vi "FPGA VI_Simulated_WithNoise_Example.vi"() -> ()   [LabVIEW 2019]
uses:
  Types/Injection.Timing.ctl
  Types/Injection.Core.Settings.ctl
  Types/Injection.Global.Settings.ctl
  Types/Injection.Mux.State.ctl
  <vilib>/Platform/TimedLoop/XDataNode/timing_clust.ctl
  <vilib>/Platform/TimedLoop/XDataNode/nitl_modes.ctl
  <vilib>/Platform/TimedLoop/XDataNode/wakeup.ctl
  Types/Injection.Core.Internal.Settings.ctl
  <vilib>/rvi/DataTransferAndStorage/Container/Common/niFpgaContainerGetUniqueNameForEmu.vi
  <vilib>/rvi/DataTransferAndStorage/Container/Common/niFpgaContainerSetEmuInfo.vi
  <vilib>/rvi/eio/common/nirviEmuReportErrorAndStop.vi
  <vilib>/rvi/Emulation/niFpgaGetClockAttributes.vi
  <vilib>/rvi/Emulation/niFpgaSctlEmulationGetInTimedLoop.vi
  <vilib>/rvi/Emulation/niFpgaEmulationReportErrorSimple.vi
  <vilib>/rvi/Memory/Memory_Emulation/nirvimemoryFastEmulation.vi
  <vilib>/rvi/Memory/Memory_Emulation/nirvimemoryEmulation.vi
  <vilib>/rvi/Emulation/niFpgaEmulationIsFPGAContextNoSignature.vi
  <vilib>/rvi/Emulation/niFpgaProcessEmulError.vi
  <vilib>/rvi/errors/nirviReportUnexpectedCaseInternalError (U32).vi
  <vilib>/rvi/Emulation/niFpgaCriticalErrorInLSC.vi
  <vilib>/rvi/DataTransferAndStorage/Container/Common/niFpgaContainerExecOnDevCompGetState.vi
  <vilib>/rvi/errors/niFpgaSetErrorForExecOnDevCompSimple.vi
  <vilib>/rvi/FIFO/Fifo_Resource/nirvififoEmulationSetSize.vi
  <vilib>/rvi/FIFO/Fifo_Resource/nirviFifoEmulationQueueMgr.vi
  <instcachedir>/0/nirviFifoEmulationQueueMgr_E5CAEC123FF24DC58D834DCA3CDAA9B5.lvgen/nirviFifoEmulationQueueMgr_E5CAEC123FF24DC58D834DCA3CDAA9B5_002.vi
  <vilib>/rvi/FIFO/Fifo_Resource/nirvififoEmulationDetermineInputValidOut.vi
  <vilib>/rvi/FIFO/Fifo_Resource/nirvififoEmulationCreateLock.vi
  <vilib>/rvi/FIFO/Fifo_Resource/nirvififoEmulationObtainLock.vi
  <vilib>/rvi/FIFO/Fifo_Resource/nirvififoEmulationReleaseLock.vi
  <vilib>/rvi/occurrence/nirviWaitOnOccurrenceBase.vi
  <vilib>/rvi/errors/nirviReportUnexpectedCaseInternalError.vi
  <vilib>/Utility/error.llb/Clear Errors.vi
  <vilib>/rvi/interface/RandomDataEmulation/niFpgaRandomDataHandleErrors.vi
  <instcachedir>/0/nirviFifoEmulationQueueMgr_E5CAEC123FF24DC58D834DCA3CDAA9B5.lvgen/nirviFifoEmulationQueueMgr_E5CAEC123FF24DC58D834DCA3CDAA9B5_001.vi
  <vilib>/rvi/LocalResourceManager/LocalResourceManager.xnode
  <vilib>/rvi/DataTransferAndStorage/Container/XNode/niFpgaContainer.xnode
  <vilib>/Platform/TimedLoop/XDataNode/XDataNode.xnode
  <vilib>/rvi/FIFO/Fifo_Resource/niFpgaFifoEmulationRefIn.vi
  <vilib>/rvi/interface/RandomDataEmulation/nirviRandomDataFpgaReadWriteTemplate.vi
  <vilib>/Platform/TimedLoop/XDataNode/XDNodeRunTimeDep.lvlib
panel:
  out "Intermediate FIFO Write Timeout":bool
  in  "Settings.Global.Injectors":T1={"Enable?"=FALSE, "Initial Voltage Threshold"=12.0, "Event Dwell Limit"=2000, "Voltage Gain"=1.0, "Current Gain"=1.0, "Filter Samples"=5, "Pretrigger Samples"=5, "Active Edge"=TRUE}
  in  "Settings.Index0.Injectors.Injector0":T2
  in  "Settings.Index1.Injectors.Injector1":T2
  in  "Settings.Index2.Injectors.Injector2":T2
  in  "Settings.Index3.Injectors.Injector3":T2
  in  "Settings.Index4.Injectors.Injector4":T2
  in  "Settings.Index5.Injectors.Injector5":T2
  in  "Settings.Timing":T3={"Injection Sample Period (Ticks)"=80}
  out "Acqusition Loop Ticks":u32
  in  "Settings.DMA":cluster{"# of Injectors":u8}={"# of Injectors"=6}
  out "Host DMA Out?":bool
  out "Intermediate Time Out?":bool
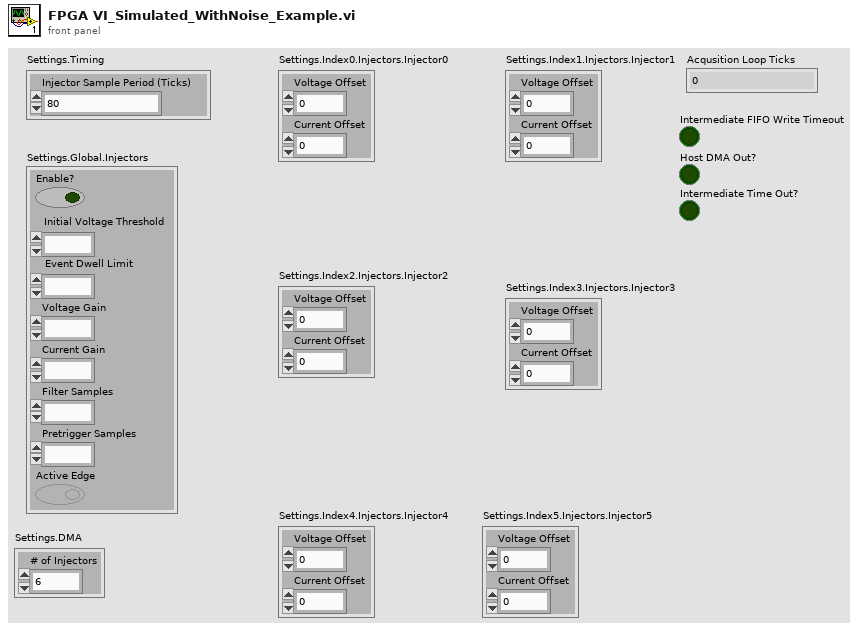
[diagram p1: front panel]
types:
  T1 = typedef "Injection.Global.Settings.ctl" = cluster{"Enable?":bool, "Initial Voltage Threshold":fxp<+/-,32,8>, "Event Dwell Limit":u16, "Voltage Gain":fxp<+/-,32,8>, "Current Gain":fxp<+/-,32,8>, "Filter Samples":u8, "Pretrigger Samples":u8, "Active Edge":bool}
  T2 = typedef "Injection.Core.Settings.ctl" = cluster{"Voltage Offset":fxp<+/-,32,8>, "Current Offset":fxp<+/-,32,8>}
  T3 = typedef "Injection.Timing.ctl" = cluster{"Injection Sample Period (Ticks)":u32}
  T4 = cluster{"Data.Samples":u32, "Injection.Period":u32, "Injector.Index":u8, "Iteration":u32}
  T5 = typedef "Injection.Mux.State.ctl" = enum8{"Wait on Transfer", "Transfer Injector Index", "Transfer # of Samples", "Transfer Injection Period", "Transfer Data Samples"}
  T6 = typedef "XDNodeRunTimeDep.lvlib/timing_clust.ctl" = cluster{"Expected End [f-1]":u64, "Actual End [f-1]":u64, "Finished Late? [f-1]":bool, "Expected End [i-1]":u64, "Actual End [i-1]":u64, "Finished Late? [i-1]":bool, "Expected Start [i]":u64, "Actual Start [i]":u64, "Expected Start [f]":u64, "Actual Start [f]":u64, "Source Name":string, "Structure Name":string, "Period":i64, "Deadline":i64, "Offset":i64, "Start":i64, "Priority":i32, "Timeout":i32, "Mode":T7, "Wakeup Reason":T8, "Error":errorcluster, "Source Type":string, "Secondary Source Type":string, "Global End Time":u64, "Global Start Time":u64, "Frame Duration":u64, "Iteration Duration":u64, "Assigned CPU":i32, "I/O Scan Engine Mode":u32}
  T7 = typedef "XDNodeRunTimeDep.lvlib/nitl_modes.ctl" = enum32{"No Change", "Process missed periods, maintain original phase", "Discard missed periods, maintain original phase", "Process missed periods, ignore original phase", "Discard missed periods, ignore original phase"}
  T8 = typedef "XDNodeRunTimeDep.lvlib/wakeup.ctl" = enum32{"Normal", "Aborted", "Asynchronous wakeup", "Timing source error", "Timed loop error", "Timeout"}
  T9 = typedef "Injection.Core.Internal.Settings.ctl" = cluster{"Data Buffer FIFO":refnum<k21>, "Capture Complete Trigger FIFO":refnum<k21>}
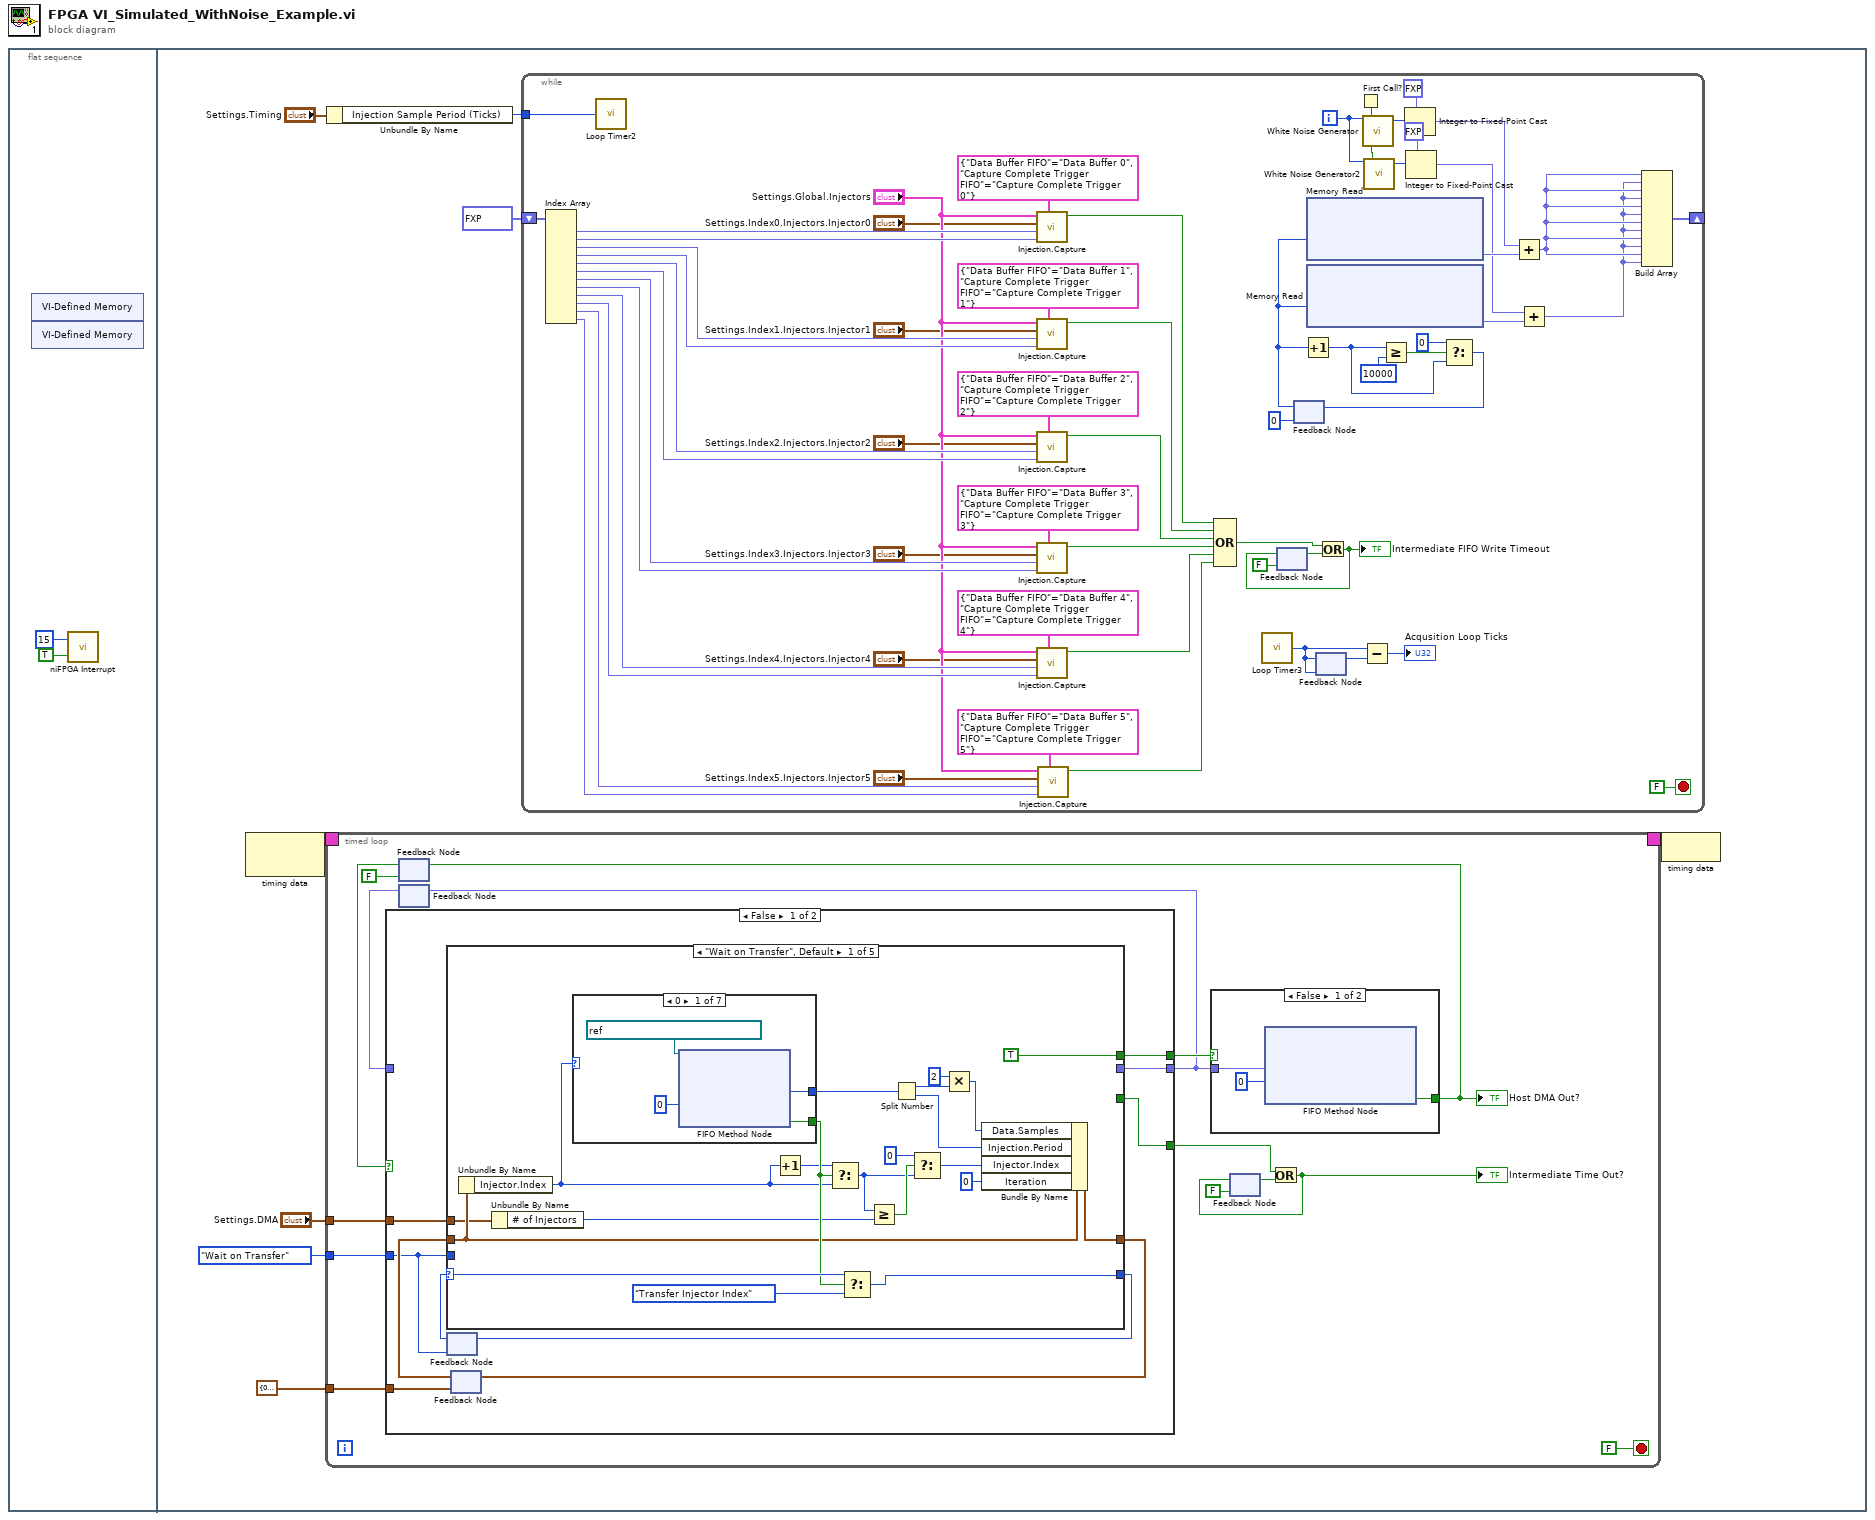
[diagram p0: block diagram]
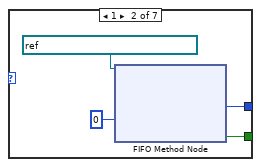
[diagram p2: hidden frame]
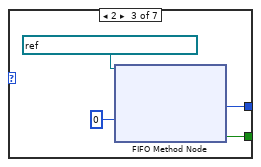
[diagram p3: hidden frame]
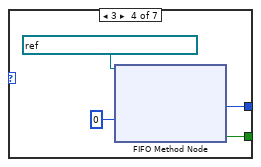
[diagram p4: hidden frame]
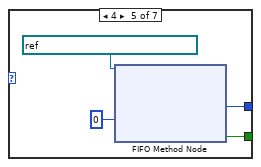
[diagram p5: hidden frame]
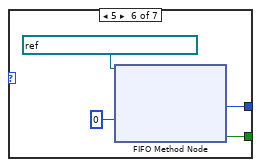
[diagram p6: hidden frame]
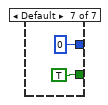
[diagram p7: hidden frame]
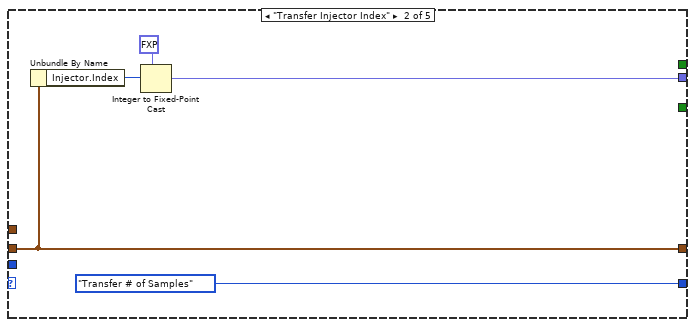
[diagram p8: hidden frame]
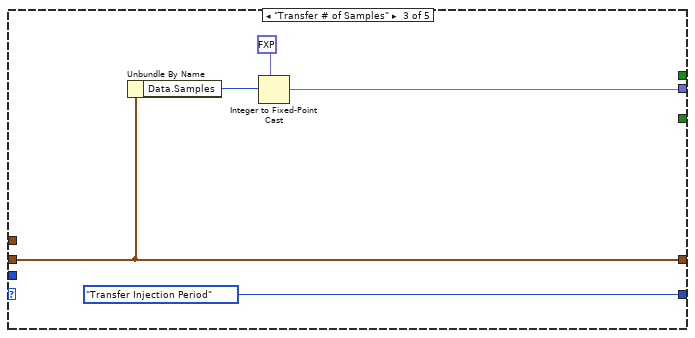
[diagram p9: hidden frame]
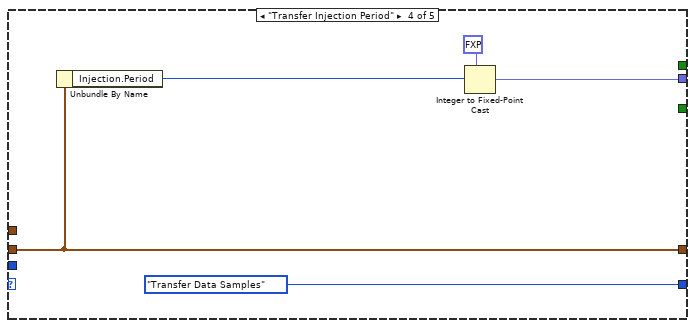
[diagram p10: hidden frame]
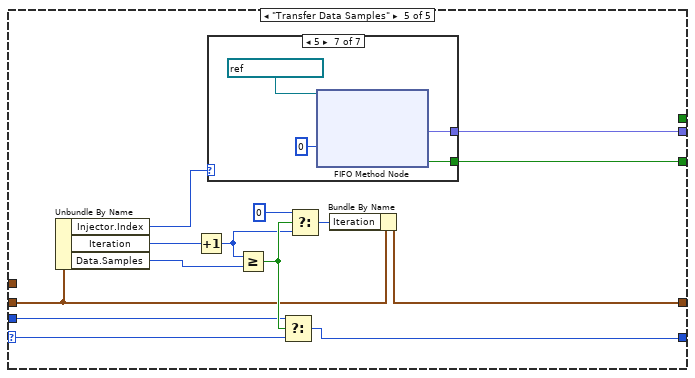
[diagram p11: hidden frame]
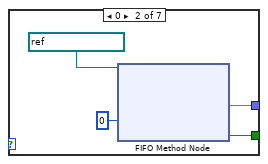
[diagram p13: hidden frame]
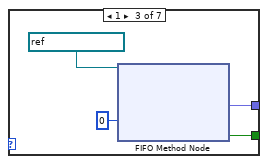
[diagram p14: hidden frame]
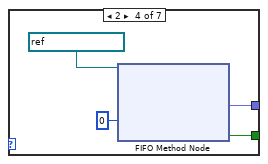
[diagram p15: hidden frame]
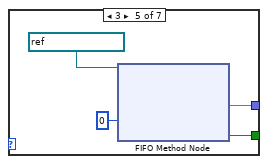
[diagram p16: hidden frame]
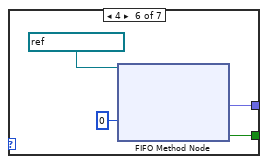
[diagram p17: hidden frame]
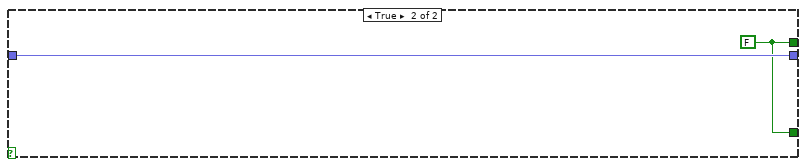
[diagram p18: hidden frame]
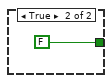
[diagram p19: hidden frame]
diagram:
  n1 = flat-sequence {
    frame #0 {
      n2 = xnode "VI-Defined Memory"() -> ()  [unwired: 1 out]
      n3 = xnode "VI-Defined Memory"() -> ()  [unwired: 1 out]
      n4 = call <vilib>:"niFPGA Interrupt.vi"("Wait Until Cleared (F)"=TRUE, "IRQ Number (0)"=u8 15) -> ()  [unwired: 1 in]
    }
    frame #1 {
      n5 = node-c288() -> (w10:T6)  [unwired: 1 in]
      n6 = timed-loop {
        timing: w10 -> [_]
        timing-out: [_] -> w9
        tunnel: "Settings.DMA" -> [w14]
        tunnel: Injection.Mux.State."Wait on Transfer" -> [w13]
        tunnel: T4 {"Data.Samples"=0, "Injection.Period"=0, "Injector.Index"=0, "Iteration"=0} ("Local.Data") -> [w12]
        stop <- FALSE stop-if-true
        n7 = feedback #1(FALSE ("Timed Out?")) -> (w22:bool)
        n8 = feedback #2() -> (w19:fxp<+/-,32,8>)  [unwired: 1 in]
        n9 = case shown="False" w22 {
          tunnel: [w34 w136] -> w20
          tunnel: [w33 w135] -> w24
          tunnel: w13 -> [w27 _]
          tunnel: [w32 w135] -> w15
          tunnel: w14 -> [w31 _]
          tunnel: w12 -> [w28 _]
          tunnel: w19 -> [_ w136]
          frame False {
            n10 = feedback #3(w27) -> (w26:T5)
            n11 = feedback #4(w28) -> (w29:T4)
            n12 = case shown="\"Wait on Transfer\", Default" w26 {
              selector: w26 -> [w55 _ _ _ w104]
              tunnel: w29 -> [w46 w85 w89 w93 w102]
              tunnel: [w54 w85 w89 w93 w101] -> w30
              tunnel: [w53 Injection.Mux.State."Transfer # of Samples" Injection.Mux.State."Transfer Injection Period" Injection.Mux.State."Transfer Data Samples" w103] -> w25
              tunnel: [_ w84 w88 w95 w100] -> w34
              tunnel: [TRUE _ _ _ _] -> w33
              tunnel: w27 -> [_ _ _ _ w97]
              tunnel: [_ _ _ _ w99] -> w32
              tunnel: w31 -> [w43 _ _ _ _]
              frame "Wait on Transfer", Default {
                n13 = Unbundle By Name(w46) -> ("Injector.Index"=w45:u8)
                n14 = Unbundle By Name(w43) -> ("# of Injectors"=w42:u8)
                n15 = case shown="0" w45 {
                  tunnel: [w58 w62 w66 w70 w74 w78 u64 0 ("Element")] -> w41
                  tunnel: [w57 w61 w65 w69 w73 w77 TRUE ("Timed Out?")] -> w51
                  frame 0 {
                    n16 = xnode ("FIFO Method Node")("Timeout"=0, "FIFO In"=refnum<k21> "Capture Complete Trigger 0") -> ("Element"=w58:u64, "Timed Out?"=w57:bool)  [unwired: 1 out]
                  }
                  frame 1 {
                    n17 = xnode ("FIFO Method Node")("Timeout"=0, "FIFO In"=refnum<k21> "Capture Complete Trigger 1") -> ("Element"=w62:u64, "Timed Out?"=w61:bool)  [unwired: 1 out]
                  }
                  frame 2 {
                    n18 = xnode ("FIFO Method Node")("Timeout"=0, "FIFO In"=refnum<k21> "Capture Complete Trigger 2") -> ("Element"=w66:u64, "Timed Out?"=w65:bool)  [unwired: 1 out]
                  }
                  frame 3 {
                    n19 = xnode ("FIFO Method Node")("Timeout"=0, "FIFO In"=refnum<k21> "Capture Complete Trigger 3") -> ("Element"=w70:u64, "Timed Out?"=w69:bool)  [unwired: 1 out]
                  }
                  frame 4 {
                    n20 = xnode ("FIFO Method Node")("Timeout"=0, "FIFO In"=refnum<k21> "Capture Complete Trigger 4") -> ("Element"=w74:u64, "Timed Out?"=w73:bool)  [unwired: 1 out]
                  }
                  frame 5 {
                    n21 = xnode ("FIFO Method Node")("Timeout"=0, "FIFO In"=refnum<k21> "Capture Complete Trigger 5") -> ("Element"=w78:u64, "Timed Out?"=w77:bool)  [unwired: 1 out]
                  }
                  frame Default {
                  }
                }
                n22 = Increment(x=w45) -> (x+1=w50:u8)
                n23 = Select(t=w50, s=w51, f=w45) -> (s? t:f=w48:u8)
                n24 = Select(t=w55, s=w51, f=Injection.Mux.State."Transfer Injector Index") -> (s? t:f=w53:T5)
                n25 = Greater Or Equal?(x=w48, y=w42) -> (x >= y?=w49:bool)
                n26 = Split Number(x=w41) -> (hi(x)=w40:u32, lo(x)=w39:u32)
                n27 = Select(t=u8 0, s=w49, f=w48) -> (s? t:f=w44:u8)
                n28 = Multiply(x=u32 2, y=w40) -> (x*y=w37:u32)
                n29 = Bundle By Name(cluster=w46, "Data.Samples"=w37, "Injection.Period"=w39, "Injector.Index"=w44, "Iteration"=u32 0) -> (w54:T4)
              }
              frame "Transfer Injector Index" {
                n30 = Unbundle By Name(w85) -> ("Injector.Index"=w86:u8)
                n31 = Integer to Fixed-Point Cast(fixed-point type=fxp<+/-,32,8> 0.0, integer=w86) -> (fixed-point=w84:fxp<+/-,32,8>)
              }
              frame "Transfer # of Samples" {
                n32 = Unbundle By Name(w89) -> ("Data.Samples"=w90:u32)
                n33 = Integer to Fixed-Point Cast(fixed-point type=fxp<+/-,32,8> 0.0, integer=w90) -> (fixed-point=w88:fxp<+/-,32,8>)
              }
              frame "Transfer Injection Period" {
                n34 = Unbundle By Name(w93) -> ("Injection.Period"=w94:u32)
                n35 = Integer to Fixed-Point Cast(fixed-point type=fxp<+/-,32,8> 0.0, integer=w94) -> (fixed-point=w95:fxp<+/-,32,8>)
              }
              frame "Transfer Data Samples" {
                n36 = Unbundle By Name(w102) -> ("Injector.Index"=w110:u8, "Iteration"=w105:u32, "Data.Samples"=w98:u32)
                n37 = Increment(x=w105) -> (x+1=w107:u32)
                n38 = case shown="5" w110 {
                  tunnel: [_ w113 w117 w121 w125 w129 w133] -> w100
                  tunnel: [_ w112 w116 w120 w124 w128 w132] -> w99
                  frame Default {
                  }
                  frame 0 {
                    n39 = xnode ("FIFO Method Node")("Timeout"=0, "FIFO In"=refnum<k21> "Data Buffer 0" ("Voltage FIFO")) -> ("Element"=w113:fxp<+/-,32,8>, "Timed Out?"=w112:bool)  [unwired: 1 out]
                  }
                  frame 1 {
                    n40 = xnode ("FIFO Method Node")("Timeout"=0, "FIFO In"=refnum<k21> "Data Buffer 1" ("Voltage FIFO")) -> ("Element"=w117:fxp<+/-,32,8>, "Timed Out?"=w116:bool)  [unwired: 1 out]
                  }
                  frame 2 {
                    n41 = xnode ("FIFO Method Node")("Timeout"=0, "FIFO In"=refnum<k21> "Data Buffer 2" ("Voltage FIFO")) -> ("Element"=w121:fxp<+/-,32,8>, "Timed Out?"=w120:bool)  [unwired: 1 out]
                  }
                  frame 3 {
                    n42 = xnode ("FIFO Method Node")("Timeout"=0, "FIFO In"=refnum<k21> "Data Buffer 3" ("Voltage FIFO")) -> ("Element"=w125:fxp<+/-,32,8>, "Timed Out?"=w124:bool)  [unwired: 1 out]
                  }
                  frame 4 {
                    n43 = xnode ("FIFO Method Node")("Timeout"=0, "FIFO In"=refnum<k21> "Data Buffer 4" ("Voltage FIFO")) -> ("Element"=w129:fxp<+/-,32,8>, "Timed Out?"=w128:bool)  [unwired: 1 out]
                  }
                  frame 5 {
                    n44 = xnode ("FIFO Method Node")("Timeout"=0, "FIFO In"=refnum<k21> "Data Buffer 5" ("Voltage FIFO")) -> ("Element"=w133:fxp<+/-,32,8>, "Timed Out?"=w132:bool)  [unwired: 1 out]
                  }
                }
                n45 = Greater Or Equal?(x=w107, y=w98) -> (x >= y?=w109:bool)
                n46 = Select(t=w97, s=w109, f=w104) -> (s? t:f=w103:T5)
                n47 = Select(t=u32 0, s=w109, f=w107) -> (s? t:f=w106:u32)
                n48 = Bundle By Name(cluster=w102, "Iteration"=w106) -> (w101:T4)
              }
            }
            n49 = feedback-in #3(w25) -> ()
            n50 = feedback-in #4(w30) -> ()
          }
          frame True {
            w135 = FALSE
          }
        }
        n51 = feedback-in #2(w20) -> ()
        n52 = case shown="False" w24 {
          tunnel: w20 -> [w138 _]
          tunnel: [w137 FALSE ("Timed Out?")] -> w23
          frame False {
            n53 = xnode ("FIFO Method Node")("Element"=w138, "Timeout"=0) -> ("Timed Out?"=w137:bool)  [unwired: 1 in, 1 out]
          }
          frame True {
          }
        }
        "Host DMA Out?" <- w23
        n54 = feedback-in #1(w23) -> ()
        n55 = feedback #5(FALSE ("Timed Out?")) -> (w17:bool)
        n56 = Or(x=w15, y=w17) -> (x .or. y?=w16:bool)
        "Intermediate Time Out?" <- w16
        n57 = feedback-in #5(w16) -> ()
      }
      n58 = Unbundle By Name("Settings.Timing") -> ("Injection Sample Period (Ticks)"=w3:u32)
      n59 = while {
        shift-right: [w156] -> _
        shift-left: fxp<+/-,24,5>[] [0.0, 0.0, 0.0, 0.0, 0.0, 0.0, 0.0, 0.0, 0.0, 0.0, 0.0, 0.0] -> [w186]
        tunnel: w3 -> [w170]
        i -> [w151]
        stop <- FALSE stop-if-true
        n60 = Index Array(array=w186) -> (element #1=w197:fxp<+/-,24,5>, element #2=w198:fxp<+/-,24,5>, element #3=w195:fxp<+/-,24,5>, element #4=w196:fxp<+/-,24,5>, element #5=w193:fxp<+/-,24,5>, element #6=w194:fxp<+/-,24,5>, element #7=w191:fxp<+/-,24,5>, element #8=w192:fxp<+/-,24,5>, element #9=w189:fxp<+/-,24,5>, element #10=w190:fxp<+/-,24,5>, element #11=w187:fxp<+/-,24,5>, element #12=w188:fxp<+/-,24,5>)  [unwired: 12 in]
        n61 = call "Loop Timer2"("Count(Ticks)"=w170) -> ()  [unwired: 1 out]
        n62 = call "Injection.Capture.vi"("FIFOs"=T9 {"Data Buffer FIFO"="Data Buffer 0", "Capture Complete Trigger FIFO"="Capture Complete Trigger 0"} ("InjectorCore.Settings"), "Current (PreScaled)"=w198, "Voltage (PreScaled)"=w197, "Settings.Index<#>.<Group>.<UserName>"="Settings.Index0.Injectors.Injector0", "Settings.Global.<Group>"="Settings.Global.Injectors") -> ("Intermediate FIFO Timeout?"=w205:bool)  [unwired: 4 in, 2 out]
        n63 = call "Injection.Capture.vi"("FIFOs"=T9 {"Data Buffer FIFO"="Data Buffer 1", "Capture Complete Trigger FIFO"="Capture Complete Trigger 1"} ("InjectorCore.Settings"), "Current (PreScaled)"=w196, "Voltage (PreScaled)"=w195, "Settings.Index<#>.<Group>.<UserName>"="Settings.Index1.Injectors.Injector1", "Settings.Global.<Group>"="Settings.Global.Injectors") -> ("Intermediate FIFO Timeout?"=w204:bool)  [unwired: 4 in, 2 out]
        n64 = call "Injection.Capture.vi"("FIFOs"=T9 {"Data Buffer FIFO"="Data Buffer 2", "Capture Complete Trigger FIFO"="Capture Complete Trigger 2"} ("InjectorCore.Settings"), "Current (PreScaled)"=w194, "Voltage (PreScaled)"=w193, "Settings.Index<#>.<Group>.<UserName>"="Settings.Index2.Injectors.Injector2", "Settings.Global.<Group>"="Settings.Global.Injectors") -> ("Intermediate FIFO Timeout?"=w203:bool)  [unwired: 4 in, 2 out]
        n65 = call "Injection.Capture.vi"("FIFOs"=T9 {"Data Buffer FIFO"="Data Buffer 3", "Capture Complete Trigger FIFO"="Capture Complete Trigger 3"} ("InjectorCore.Settings"), "Current (PreScaled)"=w192, "Voltage (PreScaled)"=w191, "Settings.Index<#>.<Group>.<UserName>"="Settings.Index3.Injectors.Injector3", "Settings.Global.<Group>"="Settings.Global.Injectors") -> ("Intermediate FIFO Timeout?"=w202:bool)  [unwired: 4 in, 2 out]
        n66 = call "Injection.Capture.vi"("FIFOs"=T9 {"Data Buffer FIFO"="Data Buffer 4", "Capture Complete Trigger FIFO"="Capture Complete Trigger 4"} ("InjectorCore.Settings"), "Current (PreScaled)"=w190, "Voltage (PreScaled)"=w189, "Settings.Index<#>.<Group>.<UserName>"="Settings.Index4.Injectors.Injector4", "Settings.Global.<Group>"="Settings.Global.Injectors") -> ("Intermediate FIFO Timeout?"=w201:bool)  [unwired: 4 in, 2 out]
        n67 = call "Injection.Capture.vi"("FIFOs"=T9 {"Data Buffer FIFO"="Data Buffer 5", "Capture Complete Trigger FIFO"="Capture Complete Trigger 5"} ("InjectorCore.Settings"), "Current (PreScaled)"=w188, "Voltage (PreScaled)"=w187, "Settings.Index<#>.<Group>.<UserName>"="Settings.Index5.Injectors.Injector5", "Settings.Global.<Group>"="Settings.Global.Injectors") -> ("Intermediate FIFO Timeout?"=w200:bool)  [unwired: 4 in, 2 out]
        n68 = Compound Arithmetic op=OR(w205, w204, w203, w202, w201, w200) -> (w175:bool)
        n69 = call "Loop Timer3"() -> ("Tick Count(Ticks)"=w171:u32)  [unwired: 1 in]
        n70 = feedback #6(FALSE ("Timed Out?")) -> (w176:bool)
        n71 = feedback #7(u32 0 ("Address")) -> (w163:u32)
        n72 = Increment(x=w163) -> (x+1=w159:u32)
        n73 = xnode ("Memory Read")("Address"=w163) -> ("Data"=w164:fxp<+/-,24,5>)  [unwired: 1 in, 1 out]
        n74 = xnode ("Memory Read")("Address"=w163) -> ("Data"=w147:fxp<+/-,24,5>)  [unwired: 1 in, 1 out]
        n75 = feedback-in #8(w171) -> ()
        n76 = feedback #8(w171) -> (w173:u32)
        n77 = Or(x=w175, y=w176) -> (x .or. y?=w174:bool)
        "Intermediate FIFO Write Timeout" <- w174
        n78 = feedback-in #6(w174) -> ()
        n79 = First Call?() -> (First Call?: T/F=w145:bool)
        n80 = Subtract(x=w171, y=w173) -> (x-y=→"Acqusition Loop Ticks":u32)
        n81 = call "White Noise Generator"("seed"=w151, "reset"=w145) -> ("white noise out"=w155:i16)  [unwired: 13 in]
        n82 = call "White Noise Generator2"("seed"=w151, "reset"=w145) -> ("white noise out"=w152:i16)  [unwired: 13 in]
        n83 = Greater Or Equal?(x=w159, y=u32 10000) -> (x >= y?=w158:bool)
        n84 = Integer to Fixed-Point Cast(fixed-point type=fxp<+/-,24,5> 0.0, integer=w155) -> (fixed-point=w150:fxp<+/-,24,5>)
        n85 = Integer to Fixed-Point Cast(fixed-point type=fxp<+/-,24,5> 0.0, integer=w152) -> (fixed-point=w148:fxp<+/-,24,5>)
        n86 = Select(t=u32 0, s=w158, f=w159) -> (s? t:f=w161:u32)
        n87 = feedback-in #7(w161) -> ()
        n88 = Add(x=w150, y=w164) -> (x+y=w149:fxp<+/-,24,5>)
        n89 = Add(x=w148, y=w147) -> (x+y=w146:fxp<+/-,24,5>)
        n90 = Build Array(w149, w146, w149, w146, w149, w146, w149, w146, w149, w146, w149, w146) -> (w156:fxp<+/-,24,5>[])
      }
      n91 = node-c288(w9) -> ()
    }
  }
